vi "Main.vi"() -> ()   [LabVIEW 2009]
panel:
  in  "Stop at target field?":bool
  out "Current Field (T)":dbl
  out "Sensor Value":dbl
  in  "Temperature":u16(ring)=1 items=["Sensor 1"=1, "Sensor 2"=2, "Sensor 3"=3]
  out "Cal file Refnum":refnum<file>
  in  "Messung Done":bool=TRUE
  out "IPS Ref":refnum<vi>
  out "Messfile Refnum":refnum<file>
  in  "Notes:":string caption="Notizen:"
  out "Measure Ref":refnum<vi>
  out "Yokogawa Ref":refnum<vi>
  in  "Stop":bool
  out "Loss":cluster{dbl, dbl}[](graph)
  out "Capacity":cluster{dbl, dbl}[](graph)
  in  "Start Kalibration":bool caption="Start"
  in  "Calibartion Settings":T1={"V/A ?"=enum."DC V", "Bias"=enum."Low", "Calibration\nB-Field (T)"=0.2, "M.time [ms]"=5000, "Delay [ms]"=500, "Start Value"=-5.0, "Target Value"=5.0, "Stepsize"=1.0} caption="Calibration Settings" {"Stepsize" min=0.0; "Delay [ms]" step=10; "M.time [ms]" step=100; "Calibration\nB-Field (T)" min=-15.0 max=15.0 step=0.1}
  in  "Calibration File":path=path "C:/Documents and Settings/memsbuddy/Desktop/Projekt/Release/Test/Test_Calibration.dat"
  in  "Start Messung":bool caption="Start"
  in  "Auto-Kalibration":bool
  in  "Measurement Settings":T2={"Start field (T)"=0.5, "Target field (T)"=-0.5, "Sweeprate (T/min)"=0.1, "Number of Sweeps"=1, "Backsweep"=TRUE, "to Zero"=TRUE, "Delay at zero"=TRUE, "Delaytime\nat zero (s)"=10, "Delay at max/min"=TRUE, "Delaytime\nmax/min (s)"=10} {"Sweeprate (T/min)" min=0.0 max=0.5 step=0.1; "Target field (T)" min=-15.0 max=15.0 step=0.1; "Start field (T)" min=-15.0 max=15.0 step=0.1}
  in  "Measurement File":path=path "C:/Documents and Settings/memsbuddy/Desktop/Projekt/Release/Test/Test.dat"
  in  "Mode":u16(ring) items=["Nanosiemens", "Dissipation-tan(delta)", "Series - KilOhms", "GigOhms", "Loss Vector"]
  in  "Deviation":u16(ring) items=["Normal", "Deviation"]
  in  "Sample name:":string
  # "(Delay must be\nswitched on)"
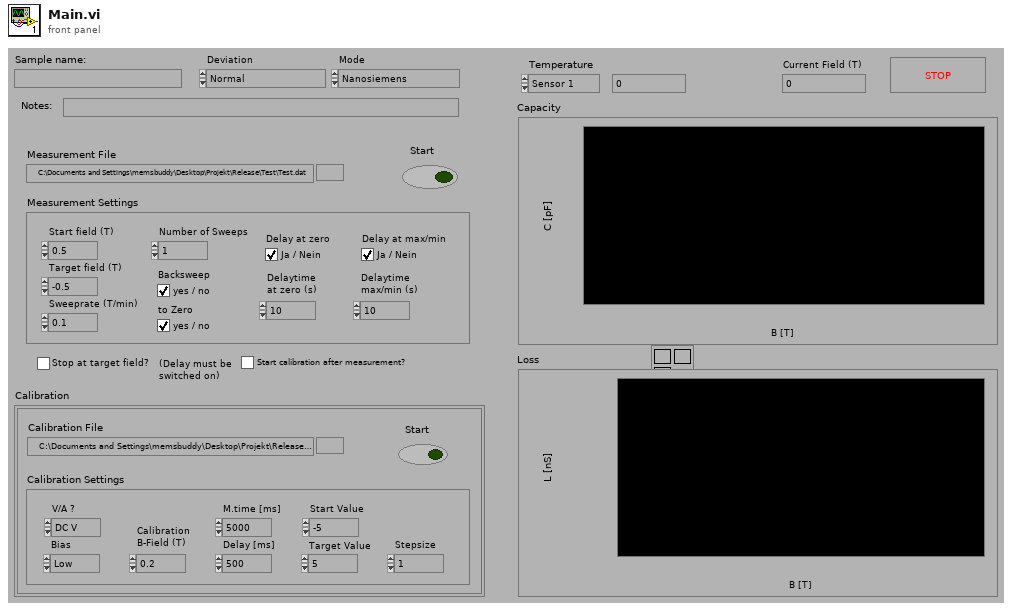
[diagram p1: front panel]
types:
  T1 = cluster{"V/A ?":enum16{"DC V", "DC A"}, "Bias":enum16{"Low", "High"}, "Calibration\nB-Field (T)":dbl, "M.time [ms]":u32, "Delay [ms]":u32, "Start Value":dbl, "Target Value":dbl, "Stepsize":dbl}
  T2 = cluster{"Start field (T)":dbl, "Target field (T)":dbl, "Sweeprate (T/min)":dbl, "Number of Sweeps":u32, "Backsweep":bool, "to Zero":bool, "Delay at zero":bool, "Delaytime\nat zero (s)":u32, "Delay at max/min":bool, "Delaytime\nmax/min (s)":u32}
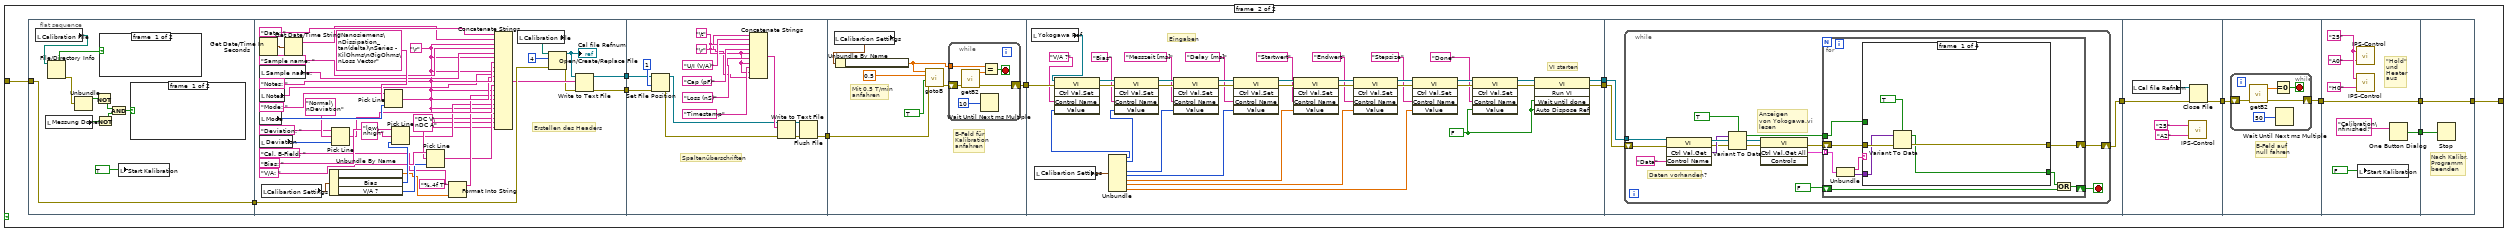
[diagram p2: hidden frame]
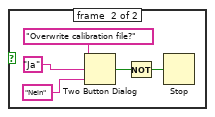
[diagram p3: hidden frame]
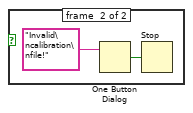
[diagram p4: hidden frame]
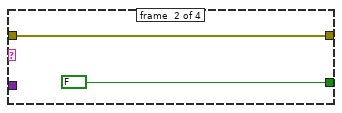
[diagram p5: hidden frame]
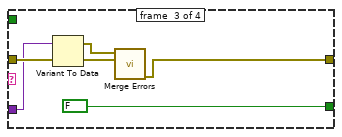
[diagram p6: hidden frame]
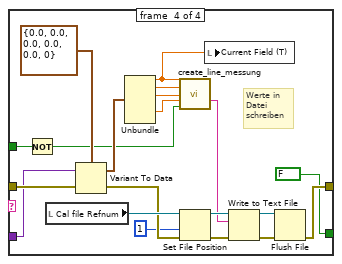
[diagram p7: hidden frame]
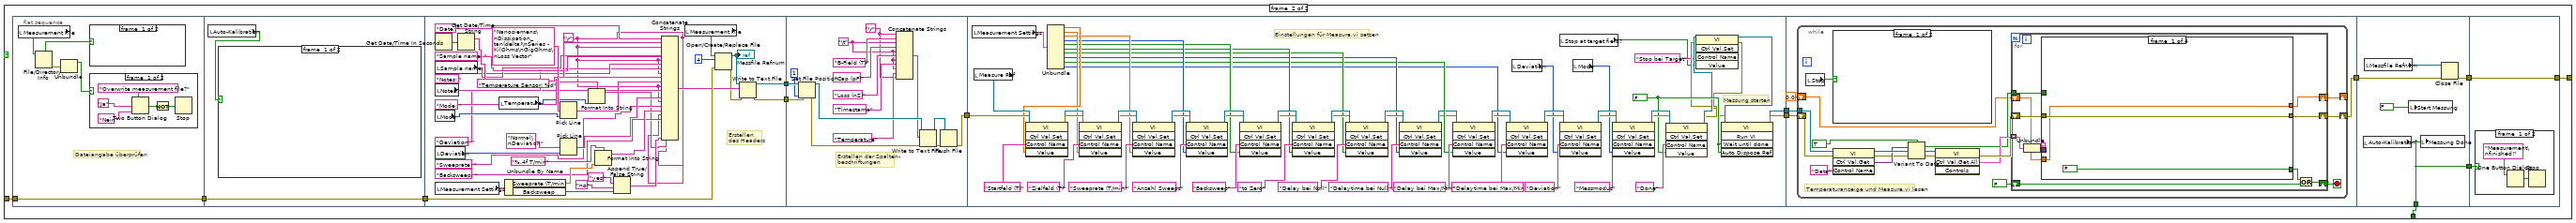
[diagram p8: hidden frame]
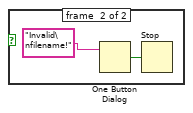
[diagram p10: hidden frame]
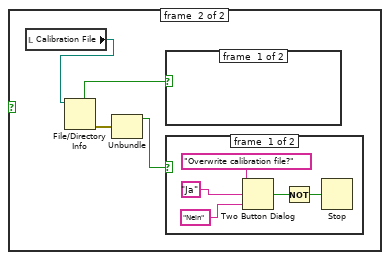
[diagram p11: hidden frame]
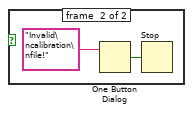
[diagram p13: hidden frame]
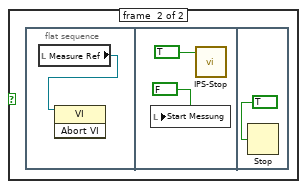
[diagram p14: hidden frame]
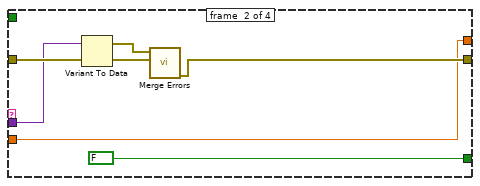
[diagram p15: hidden frame]
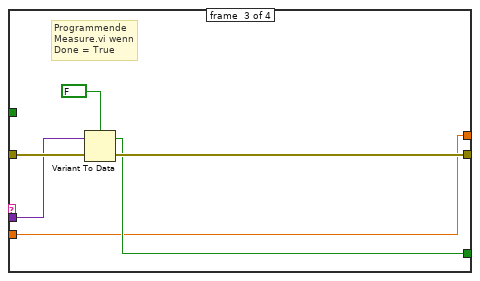
[diagram p16: hidden frame]
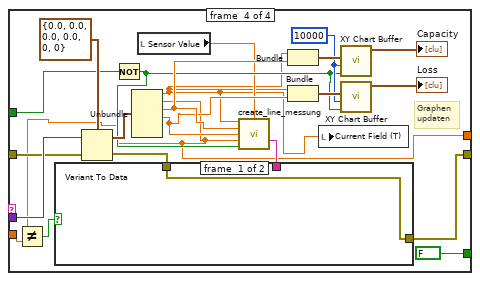
[diagram p17: hidden frame]
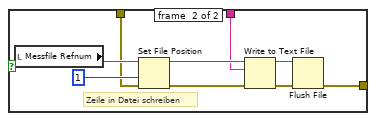
[diagram p18: hidden frame]
diagram:
  n1 = flat-sequence {
    tunnel: [w10] -> w1
    tunnel: w1 -> [w18]
    frame #0 {
      # "Funktionen werden durch lokale Variablen\nauf die Referenzen aufgerufen."
      # "VIs öffnen"
      n2 = Current VI's Path() -> (path=w17:path)
      n3 = Strip Path(path=w17) -> (stripped path=w6:path)  [unwired: 1 out]
      n4 = Build Path(base path=w6, name or relative path="Measure.vi") -> (appended path=w14:path)
      n5 = Build Path(base path=w6, name or relative path="Yokogawa.vi") -> (appended path=w13:path)
      n6 = Build Path(base path=w6, name or relative path="IPS-Control.vi") -> (appended path=w5:path)
      n7 = Open VI Reference(vi path=w14) -> (vi reference=→"Measure Ref":refnum<vi>, error out=w12:errorcluster)  [unwired: 5 in]
      n8 = Open VI Reference(vi path=w13) -> (vi reference=→"Yokogawa Ref":refnum<vi>, error out=w11:errorcluster)  [unwired: 5 in]
      n9 = Open VI Reference(vi path=w5) -> (vi reference=→"IPS Ref":refnum<vi>, error out=w4:errorcluster)  [unwired: 5 in]
      n10 = local write "Messung Done"(FALSE) -> ()
      n11 = call <vilib>:"Merge Errors.vi"("error in 3 (no error)"=w4, "error in 2 (no error)"=w11, "error in 1 (no error)"=w12) -> ("error out"=w10:errorcluster)  [unwired: 4 in]
    }
    frame #1 {
      n12 = while {
        shift-right: [w21] -> _
        shift-left: w18 -> [w22]
        stop <- FALSE stop-if-true
        n13 = event shown="[0] \"Start Messung\", \"Start Kalibration\": Value Change" {
          selector: _ -> [_ _]
          dyn-events: _ -> [_ _]
          timeout: 50 -> [_ _]
          tunnel: w22 -> [w32 w494]
          tunnel: [w28 w494] -> w21
          event #0 {
            n14 = event-data() -> ("CtlRef"=w27:refnum<vi>)  [unwired: 1 in, 5 out]
            n15 = control-ref of="Start Kalibration"() -> (w26:refnum<vi>)
            n16 = control-ref of="Start Messung"() -> (w31:refnum<vi>)
            n17 = Equal?(x=w31, y=w27) -> (x = y?=w30:bool)
            n18 = Equal?(x=w27, y=w26) -> (x = y?=w25:bool)
            n19 = case shown="True" w30 {
              tunnel: w32 -> [w248 w253]
              tunnel: [w248 w252] -> w29
              tunnel: [FALSE w251] -> w23
              frame #0 {
              }
              frame #1 {
                n20 = flat-sequence {
                  tunnel: w253 -> [w262]
                  tunnel: [w262] -> w261
                  tunnel: w261 -> [w275]
                  tunnel: [w275] -> w260
                  tunnel: w260 -> [w296]
                  tunnel: [w292] -> w259
                  tunnel: [w291] -> w258
                  tunnel: w259 -> [w339]
                  tunnel: [w326] -> w257
                  tunnel: w258 -> [w338]
                  tunnel: w257 -> [w398]
                  tunnel: [w351] -> w256
                  tunnel: [w348] -> w255
                  tunnel: w256 -> [w404]
                  tunnel: w255 -> [w403]
                  tunnel: [w402] -> w254
                  tunnel: w254 -> [w489]
                  tunnel: [w485] -> w251
                  tunnel: [w488] -> w250
                  tunnel: [w485] -> w249
                  tunnel: [w491] -> w252
                  tunnel: w250 -> [w491]
                  tunnel: w249 -> [w490]
                  frame #0 {
                    # "Dateiangabe überprüfen"
                    n21 = local read "Measurement File"() -> (w266:path)
                    n22 = File/Directory Info(path=w266) -> (directory=w264:bool, error out=w265:errorcluster)  [unwired: 1 in, 5 out]
                    n23 = Unbundle(w265) -> ("status"=w263:bool)  [unwired: 2 out]
                    n24 = case shown="False" w264 {
                      frame #0 {
                      }
                      frame #1 {
                        n25 = One Button Dialog(message="Invalid\nfilename!") -> (true=w272:bool)  [unwired: 1 in]
                        n26 = Stop(stop? (T)=w272) -> ()
                      }
                    }
                    n27 = case shown="False" w263 {
                      frame #0 {
                        n28 = Two Button Dialog(message="Overwrite measurement file?", 1:"Nein", 2:"Ja") -> (T button?=w268:bool)
                        n29 = Not(x=w268) -> (.not. x?=w267:bool)
                        n30 = Stop(stop? (T)=w267) -> ()
                      }
                      frame #1 {
                      }
                    }
                  }
                  frame #1 {
                    n31 = local read "Auto-Kalibration"() -> (w274:bool)
                    n32 = case shown="False" w274 {
                      frame #0 {
                      }
                      frame #1 {
                        n33 = local read "Calibration File"() -> (w276:path)
                        n34 = File/Directory Info(path=w276) -> (directory=w277:bool, error out=w279:errorcluster)  [unwired: 1 in, 5 out]
                        n35 = Unbundle(w279) -> ("status"=w278:bool)  [unwired: 2 out]
                        n36 = case shown="True" w277 {
                          frame #0 {
                          }
                          frame #1 {
                            n37 = One Button Dialog(message="Invalid\ncalibration\nfile!") -> (true=w285:bool)  [unwired: 1 in]
                            n38 = Stop(stop? (T)=w285) -> ()
                          }
                        }
                        n39 = case shown="False" w278 {
                          frame #0 {
                            n40 = Two Button Dialog(message="Overwrite calibration file?", 1:"Nein", 2:"Ja") -> (T button?=w281:bool)
                            n41 = Not(x=w281) -> (.not. x?=w280:bool)
                            n42 = Stop(stop? (T)=w280) -> ()
                          }
                          frame #1 {
                          }
                        }
                      }
                    }
                  }
                  frame #2 {
                    w287 = "\r"
                    # "Erstellen\ndes Headers"
                    n43 = Get Date/Time In Seconds() -> (seconds since 1Jan1904=w323:timestamp)
                    n44 = local read "Sample name:"() -> (w311:string)
                    n45 = local read "Notes:"() -> (w309:string)
                    n46 = local read "Mode"() -> (w320:u16)
                    n47 = local read "Deviation"() -> (w318:u16)
                    n48 = local read "Measurement Settings"() -> (w322:T2)
                    n49 = Get Date/Time String(seconds (now)=w323) -> (date string=w313:string)  [unwired: 2 in, 1 out]
                    n50 = local read "Temperature"() -> (w290:u16)
                    n51 = Unbundle By Name(w322) -> ("Sweeprate (T/min)"=w302:dbl, "Backsweep"=w315:bool)
                    n52 = Pick Line(multi-line string="Nanosiemens\nDissipation_tan(delta)\nSeries - KilOhms\nGigOhms\nLoss Vector", line index=w320) -> (output string=w307:string)  [unwired: 1 in]
                    n53 = Pick Line(multi-line string="Normal\nDeviation", line index=w318) -> (output string=w305:string)  [unwired: 1 in]
                    n54 = Format Into String(format string="Temperature Sensor: %d", w290) -> (resulting string=w288:string)  [unwired: 2 in, 1 out]
                    n55 = Format Into String(format string="%.4f T/min", w302) -> (resulting string=w301:string)  [unwired: 2 in, 1 out]
                    n56 = Append True/False String(1:w315, 2:"no", 3:"yes") -> (0:w299:string)  [unwired: 1 in]
                    n57 = Concatenate Strings("Date: ", w313, w287, "Sample name: ", w311, w287, "Notes: ", w309, w287, "Mode: ", w307, w287, "Deviation: ", w305, w287, "Sweeprate: ", w301, w287, "Backsweep: ", w299, w287, w288, w287, w287) -> (w294:string)
                    n58 = local read "Measurement File"() -> (w298:path)
                    n59 = Open/Create/Replace File(file path (use dialog)=w298, error in=w296, operation (0:open)=4) -> (refnum out=w295:refnum<file>, error out=w293:errorcluster)  [unwired: 3 in, 1 out]
                    "Messfile Refnum" <- w295
                    n60 = Write to Text File(file (use dialog)=w295, text=w294, error in=w293) -> (refnum out=w291:refnum<file>, error out=w292:errorcluster)  [unwired: 1 in, 1 out]
                  }
                  frame #3 {
                    w332 = "\t"
                    w324 = "\r"
                    # "Erstellen der Spalten-\nbeschriftungen"
                    n61 = Set File Position(refnum=w338, from (0:start)=1, error in=w339) -> (refnum out=w331:refnum<file>, error out=w329:errorcluster)  [unwired: 1 in]
                    n62 = Concatenate Strings(w324, "B-Field (T)", w332, "Cap (pF)", w332, "Loss (nS)", w332, "Timestamp", w332, "Temperature", w324) -> (w330:string)
                    n63 = Write to Text File(file (use dialog)=w331, text=w330, error in=w329) -> (refnum out=w327:refnum<file>, error out=w328:errorcluster)  [unwired: 1 in, 1 out]
                    n64 = Flush File(refnum=w327, error in=w328) -> (error out=w326:errorcluster)  [unwired: 1 out]
                  }
                  frame #4 {
                    w346 = FALSE
                    # "Messung starten"
                    # "Einstellungen für Measure.vi setzen"
                    n65 = local read "Measurement Settings"() -> (w399:T2)
                    n66 = local read "Measure Ref"() -> (w400:refnum<vi>)
                    n67 = Unbundle(w399) -> ("Start field (T)"=w396:dbl, "Target field (T)"=w392:dbl, "Sweeprate (T/min)"=w388:dbl, "Number of Sweeps"=w384:u32, "Backsweep"=w380:bool, "to Zero"=w376:bool, "Delay at zero"=w372:bool, "Delaytime\nat zero (s)"=w368:u32, "Delay at max/min"=w366:bool, "Delaytime\nmax/min (s)"=w360:u32)
                    n68 = invoke class="VI" method="Ctrl Val.Set"(reference=w400, error in=w398, "Control Name"="Startfeld (T)", "Value"=w396) -> (reference out=w394:refnum<vi>, error out=w395:errorcluster)  [unwired: 1 in, 3 out]
                    n69 = invoke class="VI" method="Ctrl Val.Set"(reference=w394, error in=w395, "Control Name"="Zielfeld (T)", "Value"=w392) -> (reference out=w391:refnum<vi>, error out=w390:errorcluster)  [unwired: 1 in, 3 out]
                    n70 = invoke class="VI" method="Ctrl Val.Set"(reference=w391, error in=w390, "Control Name"="Sweeprate (T/min)", "Value"=w388) -> (reference out=w387:refnum<vi>, error out=w386:errorcluster)  [unwired: 1 in, 3 out]
                    n71 = invoke class="VI" method="Ctrl Val.Set"(reference=w387, error in=w386, "Control Name"="Anzahl Sweeps", "Value"=w384) -> (reference out=w383:refnum<vi>, error out=w382:errorcluster)  [unwired: 1 in, 3 out]
                    n72 = invoke class="VI" method="Ctrl Val.Set"(reference=w383, error in=w382, "Control Name"="Backsweep", "Value"=w380) -> (reference out=w379:refnum<vi>, error out=w378:errorcluster)  [unwired: 1 in, 3 out]
                    n73 = invoke class="VI" method="Ctrl Val.Set"(reference=w379, error in=w378, "Control Name"="to Zero", "Value"=w376) -> (reference out=w375:refnum<vi>, error out=w374:errorcluster)  [unwired: 1 in, 3 out]
                    n74 = invoke class="VI" method="Ctrl Val.Set"(reference=w375, error in=w374, "Control Name"="Delay bei Null", "Value"=w372) -> (reference out=w371:refnum<vi>, error out=w370:errorcluster)  [unwired: 1 in, 3 out]
                    n75 = invoke class="VI" method="Ctrl Val.Set"(reference=w371, error in=w370, "Control Name"="Delaytime bei Null (s)", "Value"=w368) -> (reference out=w365:refnum<vi>, error out=w364:errorcluster)  [unwired: 1 in, 3 out]
                    n76 = invoke class="VI" method="Ctrl Val.Set"(reference=w365, error in=w364, "Control Name"="Delay bei Max/Min", "Value"=w366) -> (reference out=w363:refnum<vi>, error out=w362:errorcluster)  [unwired: 1 in, 3 out]
                    n77 = invoke class="VI" method="Ctrl Val.Set"(reference=w363, error in=w362, "Control Name"="Delaytime bei Max/Min (s)", "Value"=w360) -> (reference out=w358:refnum<vi>, error out=w357:errorcluster)  [unwired: 1 in, 3 out]
                    n78 = local read "Deviation"() -> (w353:u16)
                    n79 = local read "Stop at target field?"() -> (w340:bool)
                    n80 = invoke class="VI" method="Ctrl Val.Set"(reference=w358, error in=w357, "Control Name"="Deviation", "Value"=w353) -> (reference out=w356:refnum<vi>, error out=w355:errorcluster)  [unwired: 1 in, 3 out]
                    n81 = local read "Mode"() -> (w352:u16)
                    n82 = invoke class="VI" method="Ctrl Val.Set"(reference=w356, error in=w355, "Control Name"="Messmodus", "Value"=w352) -> (reference out=w350:refnum<vi>, error out=w349:errorcluster)  [unwired: 1 in, 3 out]
                    n83 = invoke class="VI" method="Ctrl Val.Set"(reference=w350, error in=w349, "Control Name"="Done", "Value"=w346) -> (reference out=w345:refnum<vi>, error out=w344:errorcluster)  [unwired: 1 in, 3 out]
                    n84 = invoke class="VI" method="Ctrl Val.Set"(reference=w345, error in=w344, "Control Name"="Stop bei Target", "Value"=w340) -> (reference out=w343:refnum<vi>, error out=w342:errorcluster)  [unwired: 1 in, 3 out]
                    n85 = invoke class="VI" method="Run VI"(reference=w343, error in=w342, "Wait until done"=w346, "Auto Dispose Ref"=w346) -> (reference out=w348:refnum<vi>, error out=w351:errorcluster)  [unwired: 1 in, 3 out]
                  }
                  frame #5 {
                    n86 = while {
                      shift-right: [w419] -> w402
                      shift-left: w404 -> [w415]
                      tunnel: w403 -> [w416]
                      shift-right: [w405] -> _
                      shift-left: 0.0 -> [w406]
                      stop <- w418 stop-if-true
                      # "Temperaturanzeige und Measure.vi lesen"
                      n87 = local read "Stop"() -> (w408:bool)
                      n88 = invoke class="VI" method="Ctrl Val.Get"(reference=w416, error in=w415, "Control Name"="Data") -> (reference out=w414:refnum<vi>, error out=w407:errorcluster, "Get Control Value Variant"=w411:variant)  [unwired: 1 in, 1 out]
                      n89 = case shown="True" w408 {
                        frame #0 {
                        }
                        frame #1 {
                          n90 = flat-sequence {
                            frame #0 {
                              n91 = local read "Measure Ref"() -> (w422:refnum<vi>)
                              n92 = invoke class="VI" method="Abort VI"(reference=w422) -> ()  [unwired: 2 in, 3 out]
                            }
                            frame #1 {
                              n93 = local write "Start Messung"(FALSE) -> ()
                              n94 = call "IPS-Stop.vi"("Stop"=TRUE) -> ()  [unwired: 1 in, 2 out]
                            }
                            frame #2 {
                              n95 = Stop(stop? (T)=TRUE) -> ()
                            }
                          }
                        }
                      }
                      n96 = Variant To Data(error in=w407, Variant=w411, type=TRUE) -> (error out=w410:errorcluster, data=w409:bool)
                      n97 = invoke class="VI" method="Ctrl Val.Get All"(reference=w414, error in=w410) -> (error out=w421:errorcluster, "Get All Control Values Variant"=w420:cluster{"Name":string, "Variant Data":variant}[])  [unwired: 2 in, 2 out]
                      n98 = for {
                        shift-right: [w432] -> w419
                        shift-left: w421 -> [w433]
                        tunnel: w420 -> [w436] mode=indexing
                        shift-right: [w431] -> w418
                        shift-left: FALSE -> [w429]
                        tunnel: w409 -> [w428]
                        shift-right: [w426] -> w405
                        shift-left: w406 -> [w427]
                        n99 = Unbundle(w436) -> ("Name"=w435:string, "Variant Data"=w434:variant)
                        n100 = case shown="\"Ausgabe-Cluster\"" w435 {
                          tunnel: w434 -> [_ w445 w451 w474]
                          tunnel: w433 -> [w439 w446 w452 w473]
                          tunnel: [w439 w442 w450 w468] -> w432
                          tunnel: [FALSE FALSE w448 FALSE] -> w430
                          tunnel: w428 -> [_ _ _ w459]
                          tunnel: [w437 w440 w447 w454] -> w426
                          tunnel: w427 -> [w437 w440 w447 w453]
                          frame #0 {
                          }
                          frame #1 {
                            n101 = Variant To Data(error in=w446, Variant=w445) -> (error out=w443:errorcluster, data=w444:errorcluster)  [unwired: 1 in]
                            n102 = call <vilib>:"Merge Errors.vi"("error in 2 (no error)"=w443, "error in 1 (no error)"=w444) -> ("error out"=w442:errorcluster)  [unwired: 5 in]
                          }
                          frame #2 {
                            # "Programmende\nMeasure.vi wenn\nDone = True"
                            n103 = Variant To Data(error in=w452, Variant=w451, type=FALSE) -> (error out=w450:errorcluster, data=w448:bool)
                          }
                          frame #3 {
                            w460 = 10000
                            # "Graphen\nupdaten"
                            n104 = Variant To Data(error in=w473, Variant=w474, type=cluster{dbl, dbl, dbl, dbl, i16, i16} {0.0, 0.0, 0.0, 0.0, 0, 0}) -> (error out=w470:errorcluster, data=w471:cluster{dbl, dbl, dbl, dbl, i16, i16})
                            n105 = Not(x=w459) -> (.not. x?=w458:bool)
                            n106 = Unbundle(w471) -> (w456:dbl, w454:dbl, w465:dbl, w464:dbl)  [unwired: 2 out]
                            n107 = Not Equal?(x=w454, y=w453) -> (x != y?=w455:bool)
                            n108 = local read "Sensor Value"() -> (w457:dbl)
                            n109 = call "create_line_messung.vi"("B-Feld"=w456, "Temperatur"=w457, "Kapazität"=w465, "Loss"=w464, "Timestamp"=w454, "Empty Line"=w458) -> ("Ausgabe"=w469:string)  [unwired: 9 in]
                            n110 = case shown="True" w455 {
                              tunnel: w470 -> [w475 w482]
                              tunnel: w469 -> [_ w479]
                              tunnel: [w475 w476] -> w468
                              frame #0 {
                              }
                              frame #1 {
                                # "Zeile in Datei schreiben"
                                n111 = local read "Messfile Refnum"() -> (w484:refnum<file>)
                                n112 = Set File Position(refnum=w484, from (0:start)=1, error in=w482) -> (refnum out=w480:refnum<file>, error out=w481:errorcluster)  [unwired: 1 in]
                                n113 = Write to Text File(file (use dialog)=w480, text=w479, error in=w481) -> (refnum out=w477:refnum<file>, error out=w478:errorcluster)  [unwired: 1 in, 1 out]
                                n114 = Flush File(refnum=w477, error in=w478) -> (error out=w476:errorcluster)  [unwired: 1 out]
                              }
                            }
                            n115 = Bundle(w456, w465) -> (w463:cluster{dbl, dbl})  [unwired: 1 in]
                            n116 = Bundle(w456, w464) -> (w461:cluster{dbl, dbl})  [unwired: 1 in]
                            n117 = local write "Current Field (T)"(w456) -> ()
                            n118 = call "XY Chart Buffer.vi"("clear first (no:F)"=w458, "chart length (points)"=w460, "new point"=w463) -> ("XY chart data"=→"Capacity":cluster{"x":dbl, "y":dbl}[])  [unwired: 8 in]
                            n119 = call "XY Chart Buffer.vi"("clear first (no:F)"=w458, "chart length (points)"=w460, "new point"=w461) -> ("XY chart data"=→"Loss":cluster{"x":dbl, "y":dbl}[])  [unwired: 8 in]
                          }
                        }
                        n120 = Or(x=w430, y=w429) -> (x .or. y?=w431:bool)
                      }
                    }
                  }
                  frame #6 {
                    n121 = local read "Auto-Kalibration"() -> (w485:bool)
                    n122 = local read "Messfile Refnum"() -> (w487:refnum<file>)
                    n123 = local write "Start Messung"(FALSE) -> ()
                    n124 = local write "Messung Done"(w485) -> ()
                    n125 = Close File(refnum=w487, error in=w489) -> (error out=w488:errorcluster)  [unwired: 1 out]
                  }
                  frame #7 {
                    n126 = case shown="False" w490 {
                      frame #0 {
                        n127 = One Button Dialog(message="Measurement\nfinished!") -> (true=w493:bool)  [unwired: 1 in]
                        n128 = Stop(stop? (T)=w493) -> ()
                      }
                      frame #1 {
                      }
                    }
                  }
                }
              }
            }
            n129 = Or(x=w23, y=w25) -> (x .or. y?=w24:bool)
            n130 = case shown="True" w24 {
              tunnel: w29 -> [w33 w37]
              tunnel: [w33 w36] -> w28
              frame #0 {
              }
              frame #1 {
                n131 = flat-sequence {
                  tunnel: w37 -> [w49]
                  tunnel: [w49] -> w47
                  tunnel: w47 -> [w70]
                  tunnel: [w66] -> w46
                  tunnel: [w65] -> w45
                  tunnel: w46 -> [w115]
                  tunnel: w45 -> [w114]
                  tunnel: [w102] -> w44
                  tunnel: w44 -> [w122]
                  tunnel: [w118] -> w43
                  tunnel: w43 -> [w165]
                  tunnel: [w137] -> w42
                  tunnel: [w130] -> w41
                  tunnel: w42 -> [w168]
                  tunnel: w41 -> [w169]
                  tunnel: [w167] -> w40
                  tunnel: w40 -> [w229]
                  tunnel: [w228] -> w39
                  tunnel: w39 -> [w231]
                  tunnel: [w232] -> w38
                  tunnel: w38 -> [w244]
                  tunnel: [w244] -> w35
                  tunnel: [w242] -> w34
                  tunnel: [w246] -> w36
                  tunnel: w35 -> [w246]
                  tunnel: w34 -> [w245]
                  frame #0 {
                    n132 = local read "Calibration File"() -> (w55:path)
                    n133 = local read "Messung Done"() -> (w53:bool)
                    n134 = File/Directory Info(path=w55) -> (directory=w56:bool, error out=w57:errorcluster)  [unwired: 1 in, 5 out]
                    n135 = Unbundle(w57) -> ("status"=w54:bool)  [unwired: 2 out]
                    n136 = Not(x=w54) -> (.not. x?=w51:bool)
                    n137 = Not(x=w53) -> (.not. x?=w52:bool)
                    n138 = case shown="True" w56 {
                      frame #0 {
                      }
                      frame #1 {
                        n139 = One Button Dialog(message="Invalid\ncalibration\nfile!") -> (true=w63:bool)  [unwired: 1 in]
                        n140 = Stop(stop? (T)=w63) -> ()
                      }
                    }
                    n141 = And(x=w51, y=w52) -> (x .and. y?=w50:bool)
                    n142 = local write "Start Kalibration"(TRUE) -> ()
                    n143 = case shown="True" w50 {
                      frame #0 {
                      }
                      frame #1 {
                        n144 = Two Button Dialog(message="Overwrite calibration file?", 1:"Nein", 2:"Ja") -> (T button?=w61:bool)
                        n145 = Not(x=w61) -> (.not. x?=w62:bool)
                        n146 = Stop(stop? (T)=w62) -> ()
                      }
                    }
                  }
                  frame #1 {
                    w73 = "\r"
                    # "Erstellen des Headers"
                    n147 = Get Date/Time In Seconds() -> (seconds since 1Jan1904=w101:timestamp)
                    n148 = local read "Sample name:"() -> (w81:string)
                    n149 = local read "Notes:"() -> (w79:string)
                    n150 = local read "Mode"() -> (w98:u16)
                    n151 = local read "Deviation"() -> (w95:u16)
                    n152 = local read "Calibartion Settings"() -> (w100:T1)
                    n153 = Get Date/Time String(seconds (now)=w101) -> (date string=w83:string)  [unwired: 2 in, 1 out]
                    n154 = Unbundle By Name(w100) -> ("Calibration\nB-Field (T)"=w86:dbl, "Bias"=w93:enum16{"Low", "High"}, "V/A ?"=w88:enum16{"DC V", "DC A"})
                    n155 = Pick Line(string ("")="Deviation: ", multi-line string="Normal\nDeviation", line index=w95) -> (output string=w77:string)
                    n156 = Pick Line(string ("")="Mode: ", multi-line string="Nanosiemens\nDissipation_tan(delta)\nSeries - KilOhms\nGigOhms\nLoss Vector", line index=w98) -> (output string=w78:string)
                    n157 = Pick Line(string ("")="Bias: ", multi-line string="low\nhigh", line index=w93) -> (output string=w75:string)
                    n158 = Pick Line(string ("")="V/A: ", multi-line string="DC V\nDC A", line index=w88) -> (output string=w74:string)
                    n159 = Format Into String(format string="%.4f T", initial string="Cal. B-Field: ", w86) -> (resulting string=w76:string)  [unwired: 1 in, 1 out]
                    n160 = Concatenate Strings("Date: ", w83, w73, "Sample name: ", w81, w73, "Notes: ", w79, w73, w78, w73, w77, w73, w76, w73, w75, w73, w74, w73, w73, w73) -> (w69:string)
                    n161 = local read "Calibration File"() -> (w72:path)
                    n162 = Open/Create/Replace File(file path (use dialog)=w72, error in=w70, operation (0:open)=4) -> (refnum out=w68:refnum<file>, error out=w67:errorcluster)  [unwired: 3 in, 1 out]
                    "Cal file Refnum" <- w68
                    n163 = Write to Text File(file (use dialog)=w68, text=w69, error in=w67) -> (refnum out=w66:refnum<file>, error out=w65:errorcluster)  [unwired: 1 in, 1 out]
                  }
                  frame #2 {
                    w109 = "\t"
                    w108 = "\r"
                    # "Spaltenüberschriften"
                    n164 = Set File Position(refnum=w115, from (0:start)=1, error in=w114) -> (refnum out=w104:refnum<file>, error out=w103:errorcluster)  [unwired: 1 in]
                    n165 = Concatenate Strings(w108, "U/I (V/A)", w109, "Cap (pF)", w109, "Loss (nS)", w109, "Timestamp", w109, w108) -> (w105:string)
                    n166 = Write to Text File(file (use dialog)=w104, text=w105, error in=w103) -> (refnum out=w106:refnum<file>, error out=w107:errorcluster)  [unwired: 1 in, 1 out]
                    n167 = Flush File(refnum=w106, error in=w107) -> (error out=w102:errorcluster)  [unwired: 1 out]
                  }
                  frame #3 {
                    # "Mit 0.5 T/min\nanfahren"
                    # "B-Feld für\nKalibration\nanfahren"
                    n168 = local read "Calibartion Settings"() -> (w123:T1)
                    n169 = Unbundle By Name(w123) -> ("Calibration\nB-Field (T)"=w119:dbl)
                    n170 = call "gotoB.vi"("error in (no error)"=w122, "Heater"=TRUE, "Sweeprate (T/min)"=0.5, "Target Field (T)"=w119) -> ("error out"=w120:errorcluster)  [unwired: 7 in]
                    n171 = while {
                      shift-right: [w128] -> w118
                      shift-left: w120 -> [w129]
                      tunnel: w119 -> [w126]
                      stop <- w125 stop-if-true
                      n172 = call "getB2.vi"("error in (no error)"=w129) -> ("error out"=w128:errorcluster, "B-Feld"=w127:dbl)  [unwired: 3 in]
                      n173 = Wait Until Next ms Multiple(millisecond multiple=10) -> ()  [unwired: 1 out]
                      n174 = Equal?(x=w126, y=w127) -> (x = y?=w125:bool)
                    }
                  }
                  frame #4 {
                    w132 = FALSE
                    # "VI starten"
                    # "Eingaben"
                    n175 = local read "Yokogawa Ref"() -> (w166:refnum<vi>)
                    n176 = local read "Calibartion Settings"() -> (w164:T1)
                    n177 = Unbundle(w164) -> ("V/A ?"=w162:enum16{"DC V", "DC A"}, "Bias"=w158:enum16{"Low", "High"}, "M.time [ms]"=w154:u32, "Delay [ms]"=w150:u32, "Start Value"=w146:dbl, "Target Value"=w142:dbl, "Stepsize"=w138:dbl)  [unwired: 1 out]
                    n178 = invoke class="VI" method="Ctrl Val.Set"(reference=w166, error in=w165, "Control Name"="V/A ?", "Value"=w162) -> (reference out=w161:refnum<vi>, error out=w160:errorcluster)  [unwired: 1 in, 3 out]
                    n179 = invoke class="VI" method="Ctrl Val.Set"(reference=w161, error in=w160, "Control Name"="Bias", "Value"=w158) -> (reference out=w157:refnum<vi>, error out=w156:errorcluster)  [unwired: 1 in, 3 out]
                    n180 = invoke class="VI" method="Ctrl Val.Set"(reference=w157, error in=w156, "Control Name"="Messzeit [ms]", "Value"=w154) -> (reference out=w153:refnum<vi>, error out=w152:errorcluster)  [unwired: 1 in, 3 out]
                    n181 = invoke class="VI" method="Ctrl Val.Set"(reference=w153, error in=w152, "Control Name"="Delay [ms]", "Value"=w150) -> (reference out=w149:refnum<vi>, error out=w148:errorcluster)  [unwired: 1 in, 3 out]
                    n182 = invoke class="VI" method="Ctrl Val.Set"(reference=w149, error in=w148, "Control Name"="Startwert", "Value"=w146) -> (reference out=w145:refnum<vi>, error out=w144:errorcluster)  [unwired: 1 in, 3 out]
                    n183 = invoke class="VI" method="Ctrl Val.Set"(reference=w145, error in=w144, "Control Name"="Endwert", "Value"=w142) -> (reference out=w141:refnum<vi>, error out=w140:errorcluster)  [unwired: 1 in, 3 out]
                    n184 = invoke class="VI" method="Ctrl Val.Set"(reference=w141, error in=w140, "Control Name"="Stepsize", "Value"=w138) -> (reference out=w136:refnum<vi>, error out=w135:errorcluster)  [unwired: 1 in, 3 out]
                    n185 = invoke class="VI" method="Ctrl Val.Set"(reference=w136, error in=w135, "Control Name"="Done", "Value"=w132) -> (reference out=w134:refnum<vi>, error out=w133:errorcluster)  [unwired: 1 in, 3 out]
                    n186 = invoke class="VI" method="Run VI"(reference=w134, error in=w133, "Wait until done"=w132, "Auto Dispose Ref"=w132) -> (reference out=w130:refnum<vi>, error out=w137:errorcluster)  [unwired: 1 in, 3 out]
                  }
                  frame #5 {
                    n187 = while {
                      tunnel: w169 -> [w177]
                      shift-right: [w171] -> w167
                      shift-left: w168 -> [w176]
                      stop <- w170 stop-if-true
                      # "Daten vorhanden?"
                      # "Anzeigen\nvon Yokogawa.vi\nlesen"
                      n188 = invoke class="VI" method="Ctrl Val.Get"(reference=w177, error in=w176, "Control Name"="Data") -> (reference out=w183:refnum<vi>, error out=w179:errorcluster, "Get Control Value Variant"=w180:variant)  [unwired: 1 in, 1 out]
                      n189 = Variant To Data(error in=w179, Variant=w180, type=TRUE) -> (error out=w178:errorcluster, data=w175:bool)
                      n190 = invoke class="VI" method="Ctrl Val.Get All"(reference=w183, error in=w178) -> (error out=w173:errorcluster, "Get All Control Values Variant"=w174:cluster{"Name":string, "Variant Data":variant}[])  [unwired: 2 in, 2 out]
                      n191 = for {
                        tunnel: w175 -> [w184]
                        tunnel: w174 -> [w192] mode=indexing
                        shift-right: [w185] -> w171
                        shift-left: w173 -> [w186]
                        shift-right: [w189] -> w170
                        shift-left: FALSE -> [w187]
                        n192 = Unbundle(w192) -> ("Name"=w191:string, "Variant Data"=w190:variant)
                        n193 = case shown="\"Ausgabe-Cluster\"" w191 {
                          tunnel: w190 -> [w195 _ w204 w224]
                          tunnel: [w193 FALSE FALSE FALSE] -> w188
                          tunnel: w186 -> [w197 w198 w205 w225]
                          tunnel: [w196 w198 w201 w208] -> w185
                          tunnel: w184 -> [_ _ _ w210]
                          frame #0 {
                            n194 = Variant To Data(error in=w197, Variant=w195, type=TRUE) -> (error out=w196:errorcluster, data=w193:bool)
                          }
                          frame #1 {
                          }
                          frame #2 {
                            n195 = Variant To Data(error in=w205, Variant=w204) -> (error out=w203:errorcluster, data=w202:errorcluster)  [unwired: 1 in]
                            n196 = call <vilib>:"Merge Errors.vi"("error in 2 (no error)"=w203, "error in 1 (no error)"=w202) -> ("error out"=w201:errorcluster)  [unwired: 5 in]
                          }
                          frame #3 {
                            # "Werte in\nDatei\nschreiben"
                            n197 = Not(x=w210) -> (.not. x?=w209:bool)
                            n198 = local read "Cal file Refnum"() -> (w218:refnum<file>)
                            n199 = Variant To Data(error in=w225, Variant=w224, type=cluster{dbl, dbl, dbl, dbl, dbl, i32} {0.0, 0.0, 0.0, 0.0, 0.0, 0}) -> (error out=w217:errorcluster, data=w222:cluster{dbl, dbl, dbl, dbl, dbl, i32})
                            n200 = Unbundle(w222) -> (w206:dbl, w221:dbl, w220:dbl, w219:dbl)  [unwired: 2 out]
                            n201 = call "create_line_messung.vi"("B-Feld"=w206, "Kapazität"=w221, "Loss"=w220, "Timestamp"=w219, "Empty Line"=w209) -> ("Ausgabe"=w213:string)  [unwired: 10 in]
                            n202 = Set File Position(refnum=w218, from (0:start)=1, error in=w217) -> (refnum out=w215:refnum<file>, error out=w214:errorcluster)  [unwired: 1 in]
                            n203 = local write "Current Field (T)"(w206) -> ()
                            n204 = Write to Text File(file (use dialog)=w215, text=w213, error in=w214) -> (refnum out=w211:refnum<file>, error out=w212:errorcluster)  [unwired: 1 in, 1 out]
                            n205 = Flush File(refnum=w211, error in=w212) -> (error out=w208:errorcluster)  [unwired: 1 out]
                          }
                        }
                        n206 = Or(x=w188, y=w187) -> (x .or. y?=w189:bool)
                      }
                    }
                  }
                  frame #6 {
                    n207 = local read "Cal file Refnum"() -> (w230:refnum<file>)
                    n208 = call "IPS-Control.vi"("Frage"="A2", "address string"="25") -> ()  [unwired: 1 out]
                    n209 = Close File(refnum=w230, error in=w229) -> (error out=w228:errorcluster)  [unwired: 1 out]
                  }
                  frame #7 {
                    # "B-Feld auf\nnull fahren"
                    n210 = while {
                      shift-right: [w236] -> w232
                      shift-left: w231 -> [w237]
                      stop <- w234 stop-if-true
                      n211 = call "getB2.vi"("error in (no error)"=w237) -> ("error out"=w236:errorcluster, "B-Feld"=w235:dbl)  [unwired: 3 in]
                      n212 = Equal To 0?(x=w235) -> (x = 0?=w234:bool)
                      n213 = Wait Until Next ms Multiple(millisecond multiple=50) -> ()  [unwired: 1 out]
                    }
                  }
                  frame #8 {
                    w240 = "25"
                    # "\"Hold\"\nund\nHeater\naus"
                    n214 = call "IPS-Control.vi"("Frage"="A0", "address string"=w240) -> ()  [unwired: 1 out]
                    n215 = call "IPS-Control.vi"("Frage"="H0", "address string"=w240) -> ()  [unwired: 1 out]
                    n216 = local write "Start Kalibration"(FALSE) -> ()
                    n217 = One Button Dialog(message="Calibration\nfinished!") -> (true=w242:bool)  [unwired: 1 in]
                  }
                  frame #9 {
                    # "Nach Kalibr.\nProgramm\nbeenden"
                    n218 = Stop(stop? (T)=w245) -> ()
                  }
                }
              }
            }
          }
          event #1 {
            n219 = event-data() -> ()  [unwired: 1 in, 3 out]
          }
        }
      }
    }
  }
